vi "Parse Buttons.vi"(11 "stream in":u8[](array[numeric])) -> (0 "Buttons":T1, 3 "stream out":u8[](array[numeric]))   [LabVIEW 2013]
doc: "Read the status of cargo bay buttons from a UART stream."
uses:
  Buttons.ctl
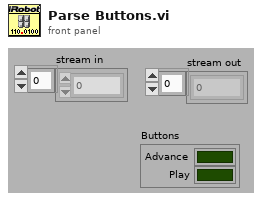
[diagram p1: front panel]
types:
  T1 = typedef "Buttons.ctl" = cluster{"Advance":bool, "Play":bool}
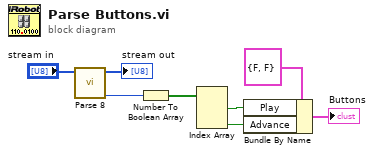
[diagram p0: block diagram]
diagram:
  n1 = call "Parse 8.vi"("stream in"="stream in") -> ("value"=w1:u8, "stream out"=→"stream out":u8[])  [unwired: 9 out]
  n2 = Number To Boolean Array(number=w1) -> (Boolean array=w8:bool[])
  n3 = Index Array(array=w8) -> (element #1=w6:bool, element #3=w5:bool)  [unwired: 3 in, 1 out]
  n4 = Bundle By Name(cluster=T1 {"Advance"=FALSE, "Play"=FALSE} ("Buttons"), "Play"=w6, "Advance"=w5) -> (→"Buttons":T1)
